vi "TB-Stop.vi"(0 "state in":T3, 1 "Log in":T1, 11 "error in (no error)":errorcluster, 13 "Queue in":T6) -> (3 "Log out":T1, 4 "state out":T3, 8 "Finished":bool, 15 "error out":errorcluster)   [LabVIEW 2020]
uses:
  Typedefs/TB-Mic Queue.ctl
  Typedefs/TB-Runtime state.ctl
  <vilib>/sound2/lvsound2.llb/Sound File Refnum.ctl
  Typedefs/TB-Setup Log.ctl
  Typedefs/TB-Log.ctl
  Typedefs/TB-Slack State.ctl
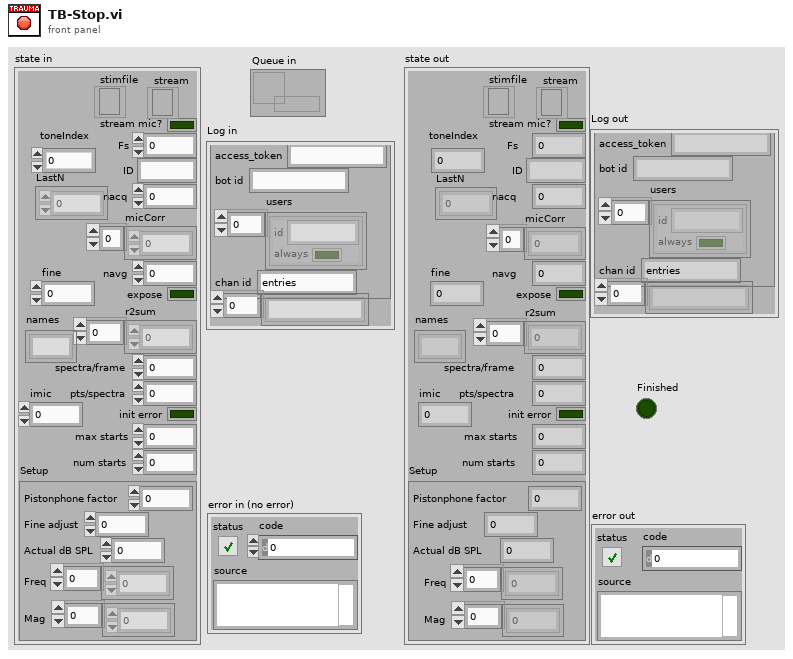
[diagram p1: front panel]
types:
  T1 = typedef "TB-Log.ctl" = cluster{"Slack":T2, "entries":string[]}
  T2 = typedef "TB-Slack State.ctl" = cluster{"access_token":string, "bot id":string, "users":cluster{"id":string, "always":bool}[], "chan id":string}
  T3 = typedef "TB-Runtime state.ctl" = cluster{"stimfile":T4, "stream mic?":bool, "Fs":dbl, "ID":string, "micCorr":dbl[], "navg":i32, "r2sum":dbl[], "expose":bool, "spectra/frame":i32, "pts/spectra":i32, "nacq":i32, "init error":bool, "max starts":i32, "num starts":i32, "Setup":T5, "toneIndex":i32, "LastN":dbl[], "fine":dbl, "imic":i32, "stream":refnum<file>, "names":string[]}
  T4 = typedef "Sound File Refnum.ctl" = refnum<file>
  T5 = typedef "TB-Setup Log.ctl" = cluster{"Pistonphone factor":dbl, "Fine adjust":dbl, "Actual dB SPL":dbl, "Freq":dbl[], "Mag":dbl[]}
  T6 = typedef "TB-Mic Queue.ctl" = refnum<queue>
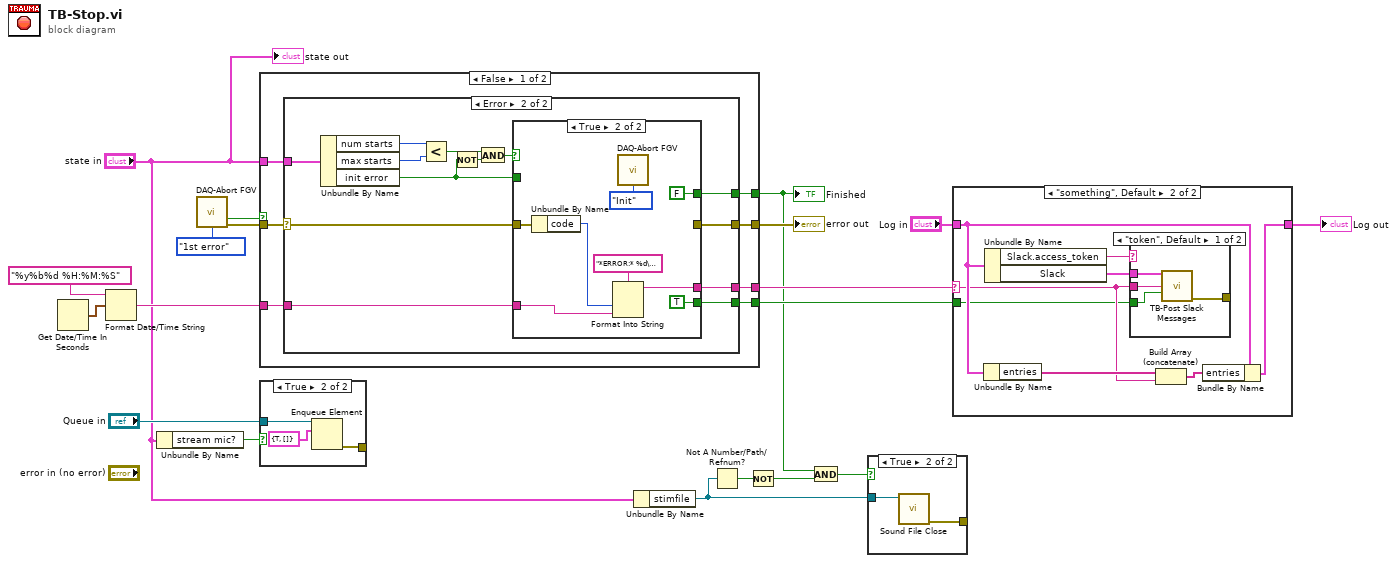
[diagram p0: block diagram]
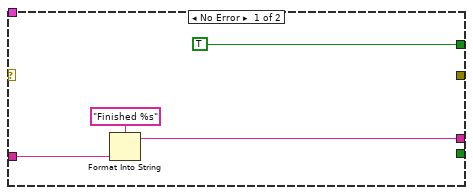
[diagram p4: hidden frame]
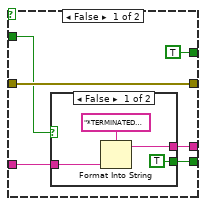
[diagram p5: hidden frame]
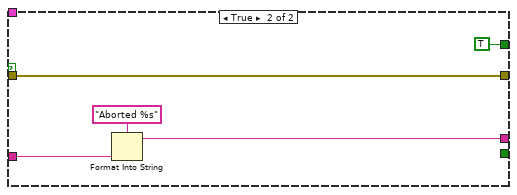
[diagram p7: hidden frame]
diagram:
  n1 = Get Date/Time In Seconds() -> (seconds since 1Jan1904=w13:timestamp)
  n2 = Format Date/Time String(time format string (%c)="%y%b%d %H:%M:%S", seconds (now)=w13) -> (date/time string=w11:string)  [unwired: 1 in]
  n3 = Unbundle By Name("state in") -> ("stream mic?"=w19:bool)
  n4 = call "DAQ-Abort FGV.vi"("Action"=enum16{"Default", "Init", "Abort", "1st error"}."1st error") -> ("Was aborted"=w16:bool, "Errors"=w15:errorcluster)  [unwired: 12 in, 1 out]
  n5 = case shown="False" w16 {
    tunnel: "state in" -> [w26 _]
    tunnel: w15 -> [w25 w66]
    tunnel: [w23 w66] -> w14
    tunnel: [w24 TRUE] -> w5
    tunnel: w11 -> [w22 w65]
    tunnel: [w21 w63] -> w8
    tunnel: [w20 _] -> w6
    frame False {
      n6 = case shown="Error" w25 {
        selector: w25 -> [_ w36]
        tunnel: w26 -> [_ w43]
        tunnel: [TRUE w34] -> w24
        tunnel: [_ w35] -> w23
        tunnel: w22 -> [w28 w33]
        tunnel: [w27 w32] -> w21
        tunnel: [_ w31] -> w20
        frame No Error {
          n7 = Format Into String(format string="Finished %s", w28) -> (resulting string=w27:string)  [unwired: 2 in, 1 out]
        }
        frame Error {
          n8 = Unbundle By Name(w43) -> ("num starts"=w42:i32, "max starts"=w41:i32, "init error"=w38:bool)
          n9 = Less?(x=w42, y=w41) -> (x < y?=w40:bool)
          n10 = Not(x=w38) -> (.not. x?=w37:bool)
          n11 = And(x=w40, y=w37) -> (x .and. y?=w39:bool)
          n12 = case shown="True" w39 {
            tunnel: w38 -> [w47 _]
            tunnel: w36 -> [w49 w61]
            tunnel: [w49 _] -> w35
            tunnel: [TRUE FALSE] -> w34
            tunnel: w33 -> [w46 w57]
            tunnel: [w45 w59] -> w32
            tunnel: [w44 TRUE] -> w31
            frame False {
              n13 = case shown="False" w47 {
                tunnel: w46 -> [w52 _]
                tunnel: [w51 _] -> w45
                tunnel: [TRUE _] -> w44
                frame False {
                  n14 = Format Into String(format string="*TERMINATED WITH ERROR* %s\n", w52) -> (resulting string=w51:string)  [unwired: 2 in, 1 out]
                }
                frame True {
                }
              }
            }
            frame True {
              n15 = Unbundle By Name(w61) -> ("code"=w58:i32)
              n16 = Format Into String(format string="*ERROR:* %d\nRestarting %s\n", w58, w57) -> (resulting string=w59:string)  [unwired: 2 in, 1 out]
              n17 = call "DAQ-Abort FGV.vi"("Action"=enum16{"Default", "Init", "Abort", "1st error"}."Init") -> ()  [unwired: 12 in, 3 out]
            }
          }
        }
      }
    }
    frame True {
      n18 = Format Into String(format string="Aborted %s", w65) -> (resulting string=w63:string)  [unwired: 2 in, 1 out]
    }
  }
  "error out" <- w14
  "Finished" <- w5
  n19 = case shown="True" w19 {
    tunnel: "Queue in" -> [_ w69]
    tunnel: [_ w68] -> _
    frame False {
    }
    frame True {
      n20 = Enqueue Element(queue=w69, element=cluster{bool, dbl[][]} {TRUE, []}) -> (error out=w68:errorcluster)  [unwired: 2 in, 2 out]
    }
  }
  n21 = Unbundle By Name("state in") -> ("stimfile"=w3:T4)
  n22 = Not A Number/Path/Refnum?(number/path/refnum=w3) -> (NaN/Path/Refnum?=w2:bool)
  n23 = Not(x=w2) -> (.not. x?=w1:bool)
  n24 = And(x=w5, y=w1) -> (x .and. y?=w4:bool)
  n25 = case shown="True" w4 {
    tunnel: w3 -> [_ w71]
    tunnel: [_ w70] -> _
    frame False {
    }
    frame True {
      n26 = call <vilib>:"Sound File Close.vi"("sound file refnum"=w71) -> ("error out"=w70:errorcluster)  [unwired: 10 in]
    }
  }
  n27 = case shown="\"something\", Default" w8 {
    selector: w8 -> [_ w74]
    tunnel: "Log in" -> [w72 w77]
    tunnel: [w72 w80] -> w9
    tunnel: w6 -> [_ w73]
    frame "" {
    }
    frame "something", Default {
      n28 = Unbundle By Name(w77) -> ("entries"=w79:string[])
      n29 = Unbundle By Name(w77) -> ("Slack.access_token"=w76:string, "Slack"=w75:T2)
      n30 = case shown="\"token\", Default" w76 {
        tunnel: w75 -> [w84 _]
        tunnel: w74 -> [w83 _]
        tunnel: [w82 _] -> _
        tunnel: w73 -> [w81 _]
        frame "token", Default {
          n31 = call "TB-Post Slack Messages.vi"("Slack"=w84, "Message"=w83, "error notification (F)"=w81) -> ("error out"=w82:errorcluster)  [unwired: 12 in]
        }
        frame "" {
        }
      }
      n32 = Build Array (concatenate)(w79, w74) -> (w78:string[])
      n33 = Bundle By Name(cluster=w77, "entries"=w78) -> (w80:T1)
    }
  }
  "Log out" <- w9
  "state out" <- "state in"
